vi "PDLM_GetLHCurrentTemp.vi"(8 "error in (no error)":errorcluster, 10 "ScaleID":T1, 11 "USBIdx":i32) -> (0 "error out":errorcluster, 2 "CurrTemp":sgl, 3 "return type":i32)   [LabVIEW 2017]
uses:
  PDLM_ScaleID.ctl
  PDLM_DllPath_global.vi
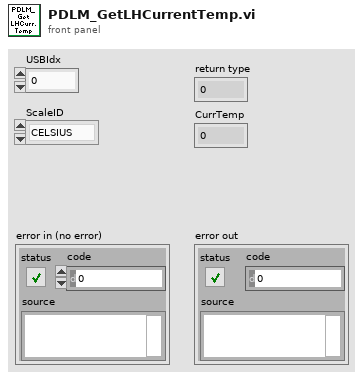
[diagram p1: front panel]
types:
  T1 = typedef "PDLM_ScaleID.ctl" = enum32{"CELSIUS", "FAHRENHEIT", "KELVIN"}
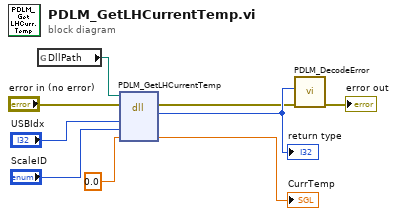
[diagram p0: block diagram]
diagram:
  n1 = global read "PDLM_DllPath_global.vi" "DllPath"() -> (w5:path)
  n2 = dll-call lib="M:/_dev/progs/LabVIEW/_lib/PQ/Taiko/pdlm_lib.dll" fn="PDLM_GetLHCurrentTemp"(path in=w5, error in="error in (no error)", "USBIdx"="USBIdx", "ScaleID"="ScaleID", "CurrTemp"=sgl 0.0 ("mode")) -> (error out=w7:errorcluster, "return type"=w8:i32, "CurrTemp"=→"CurrTemp":sgl)  [unwired: 3 in, 1 out]
  "return type" <- w8
  n3 = call "PDLM_DecodeError.vi"("error in (no error)"=w7, "code"=w8) -> ("error out"=→"error out":errorcluster)  [unwired: 7 in, 2 out]
